vi "ReadTempSensorParam332.vi"(0 "Nom":string, 1 "Error in":errorcluster) -> (2 "Configurations":string[](array[string]), 3 "SensorPar":T1={"TableTC"=1, "TableConv"=1, "Compensation"=1, "Type"=9} caption="Paramètre de configuration d'entrée" {"Compensation" items=["Off", "On"]; "TableConv" max=60 step=1; "Type" items=["Silicon Diode", "GaAlAs Diode", "Platinum 100 (250 Ohms)", "Platinum 100 (500 Ohms)", "Platinum 1000 Ohms", "NTC RTD 75mV 7.5 KOhms", "Thermocouple 25mV", "Thermocouple 50mV", "NTC RTD 75mV 75 Ohms", "NTC RTD 75mV 750 Ohms", "NTC RTD 75mV 7.5 KOhms", "NTC RTD 75mV 75 KOhms", "NTC RTD 75mV Auto"]; "TableTC" max=41 step=1}, 5 "Error out":errorcluster)   [LabVIEW 2012]
doc: "Ce VI ouvre le fichier de sauvegarde des modèles de configuration et lit les valeurs du modèle spécifié."
uses:
  <userlib>/LSCI 332/LSCI332.llb/InConfigPar332.ctl
  <vilib>/Utility/config.llb/Read Key (I32).vi
  <vilib>/Utility/config.llb/NI_LVConfig.lvlib
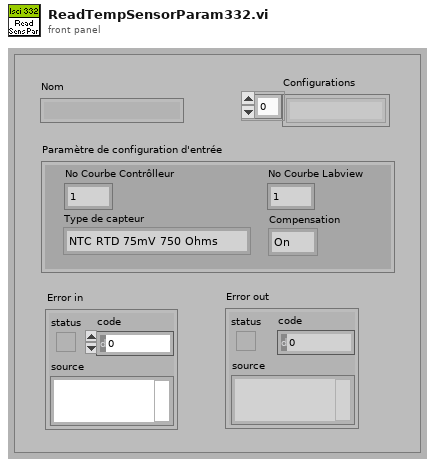
[diagram p1: front panel]
types:
  T1 = typedef "InConfigPar332.ctl" = cluster{"TableTC":u16, "TableConv":u16, "Compensation":u16, "Type":u16}
  T2 = typedef "NI_LVConfig.lvlib/Config Data RefNum.ctl" = refnum<k1>
  T3 = cluster{"[0]":u16, "[1]":u16, "[2]":u16, "[3]":u16, "[4]":u16, "[5]":u16, "[6]":u16, "[7]":u16, "[8]":u16}
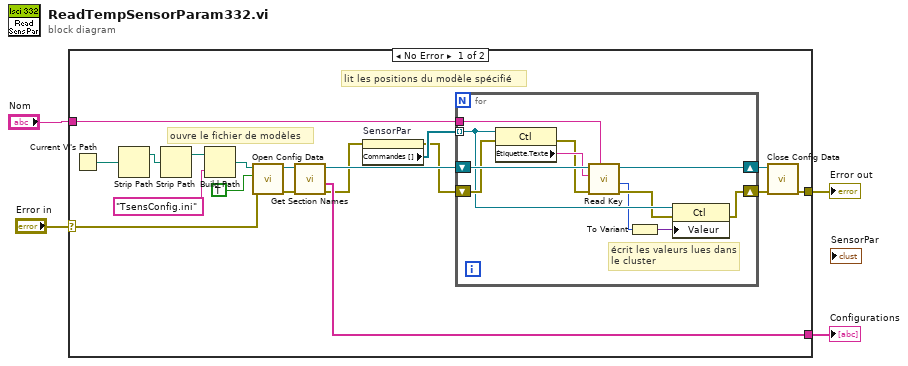
[diagram p0: block diagram]
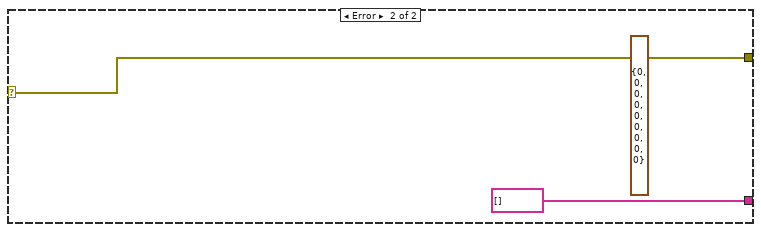
[diagram p2: hidden frame]
diagram:
  n1 = case shown="No Error" "Error in" {
    selector: "Error in" -> [w17 w35]
    tunnel: "Nom" -> [w12 _]
    tunnel: [w18 w35] -> w4
    tunnel: [w14 string[] [] ("section names")] -> w1
    frame No Error {
      # "lit les positions du modèle spécifié"
      # "ouvre le fichier de modèles"
      n2 = Current VI's Path() -> (path=w21:path)
      n3 = Strip Path(path=w21) -> (stripped path=w6:path)  [unwired: 1 out]
      n4 = Strip Path(path=w6) -> (stripped path=w5:path)  [unwired: 1 out]
      n5 = Build Path(base path=w5, name or relative path="TsensConfig.ini") -> (appended path=w19:path)
      n6 = call <vilib>:"Open Config Data.vi"("error in (no error)"=w17, "create file if necessary (T)"=TRUE ("create file if necessary? (T)"), "configuration file path"=w19) -> ("error out"=w16:errorcluster, "refnum"=w15:T2)  [unwired: 6 in, 1 out]
      n7 = call <vilib>:"Get Section Names.vi"("error in (no error)"=w16, "refnum"=w15) -> ("error out"=w8:errorcluster, "section names"=w14:string[], "refnum out"=w13:T2)  [unwired: 7 in]
      n8 = property on="SensorPar" class="Clust (strict)"(error in=w8) -> (error out=w7:errorcluster, "Commandes []"=w9:refnum<vi>[])  [unwired: 1 in, 1 out]
      n9 = for {
        shift-right: [w33] -> w11
        shift-left: w13 -> [w32]
        shift-right: [w25] -> w10
        shift-left: w7 -> [w29]
        tunnel: w12 -> [w30]
        tunnel: w9 -> [w27] mode=indexing
        # "écrit les valeurs lues dans le cluster"
        n10 = property class="Ctl"(reference=w27, error in=w29) -> (error out=w28:errorcluster, "Étiquette.Texte"=w31:string)  [unwired: 1 out]
        n11 = call-poly <vilib>:"Read Key.vi"("section"=w30, "error in (no error)"=w28, "key"=w31, "refnum"=w32) -> ("error out"=w26:errorcluster, "value"=w23:i32, "refnum out"=w33:T2)  [unwired: 4 in, 1 out]
        n12 = To Variant(anything=w23) -> (Variant=w24:variant)
        n13 = property class="Ctl"(reference=w27, error in=w26, "Valeur"=w24) -> (error out=w25:errorcluster)  [unwired: 1 out]
      }
      n14 = call <vilib>:"Close Config Data.vi"("error in (no error)"=w10, "refnum"=w11) -> ("error out"=w18:errorcluster)  [unwired: 8 in, 1 out]
    }
    frame Error {
      (unwired) T3 {"[0]"=0, "[1]"=0, "[2]"=0, "[3]"=0, "[4]"=0, "[5]"=0, "[6]"=0, "[7]"=0, "[8]"=0}
    }
  }
  "Error out" <- w4
  "Configurations" <- w1
